vi "overwritePos.vi"(2 "overwrite angle":bool, 3 "Source":u16(ring) items=["Odometry", "Lidar"], 4 "lidarPosInput":cluster{"xPos":dbl, "yPos":dbl, "Theta":dbl}, 5 "odomPosInput":cluster{"xPos":dbl, "yPos":dbl, "Theta":dbl}) -> (1 "posOutput":cluster{"xPos":dbl, "yPos":dbl, "Theta":dbl})   [LabVIEW 2016]
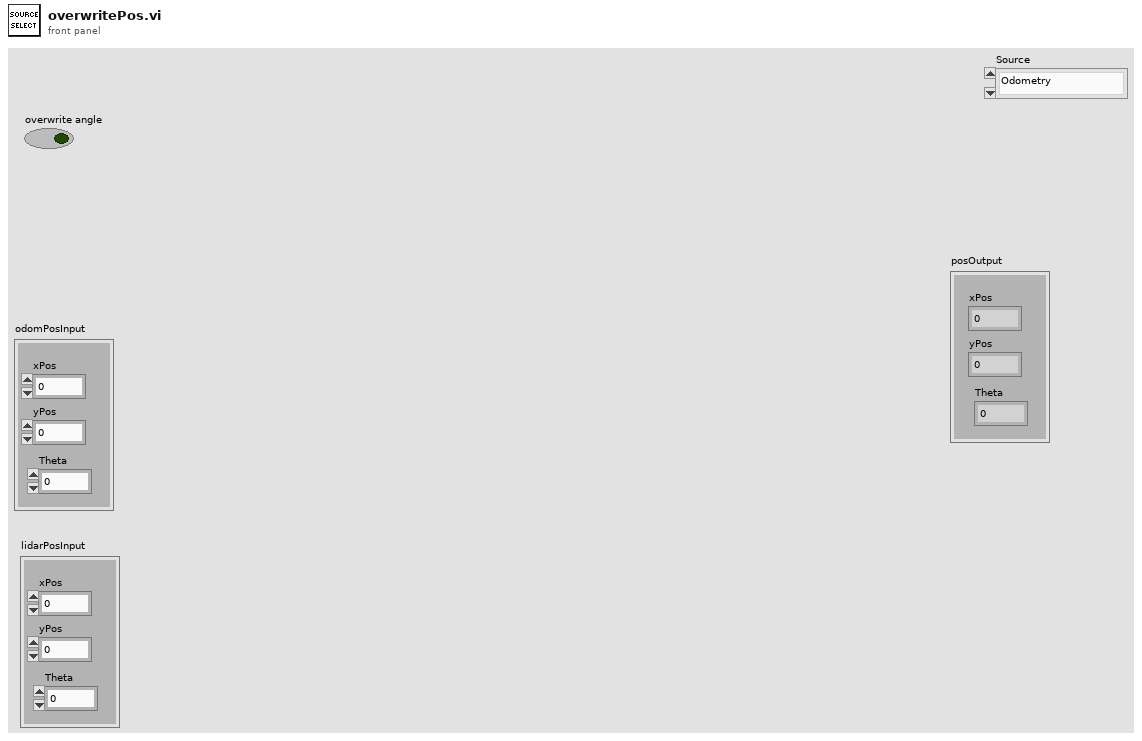
[diagram p1: front panel]
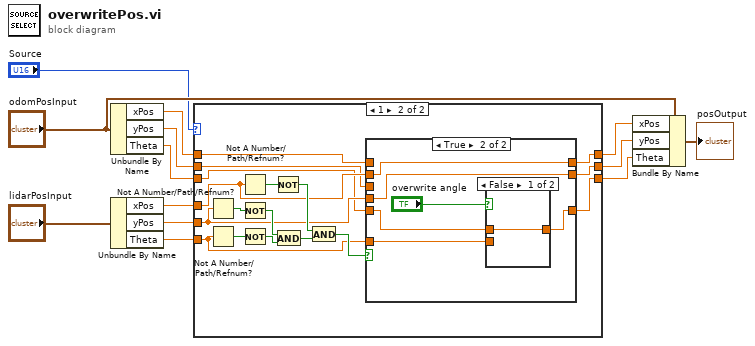
[diagram p0: block diagram]
diagram:
  n1 = Unbundle By Name("odomPosInput") -> ("xPos"=w5:dbl, "yPos"=w4:dbl, "Theta"=w1:dbl)
  n2 = Unbundle By Name("lidarPosInput") -> ("xPos"=w3:dbl, "yPos"=w7:dbl, "Theta"=w2:dbl)
  n3 = case shown="1" "Source" {
    tunnel: [w16 w25] -> w12
    tunnel: w5 -> [w16 w19]
    tunnel: [w15 w23] -> w11
    tunnel: w4 -> [w15 w18]
    tunnel: [w14 w21] -> w10
    tunnel: w1 -> [w14 w17]
    tunnel: w3 -> [_ w24]
    tunnel: w7 -> [_ w22]
    tunnel: w2 -> [_ w20]
    frame 0, Default {
    }
    frame 1 {
      n4 = Not A Number/Path/Refnum?(number/path/refnum=w22) -> (NaN/Path/Refnum?=w32:bool)
      n5 = Not A Number/Path/Refnum?(number/path/refnum=w20) -> (NaN/Path/Refnum?=w33:bool)
      n6 = Not A Number/Path/Refnum?(number/path/refnum=w24) -> (NaN/Path/Refnum?=w31:bool)
      n7 = Not(x=w32) -> (.not. x?=w30:bool)
      n8 = Not(x=w33) -> (.not. x?=w29:bool)
      n9 = Not(x=w31) -> (.not. x?=w27:bool)
      n10 = And(x=w30, y=w29) -> (x .and. y?=w28:bool)
      n11 = And(x=w27, y=w28) -> (x .and. y?=w26:bool)
      n12 = case shown="True" w26 {
        tunnel: [w36 w42] -> w25
        tunnel: w24 -> [_ w42]
        tunnel: [w35 w41] -> w23
        tunnel: w22 -> [_ w41]
        tunnel: [w34 w40] -> w21
        tunnel: w20 -> [_ w38]
        tunnel: w19 -> [w36 _]
        tunnel: w18 -> [w35 _]
        tunnel: w17 -> [w34 w39]
        frame False {
        }
        frame True {
          n13 = case shown="False" "overwrite angle" {
            tunnel: [w43 w44] -> w40
            tunnel: w38 -> [_ w44]
            tunnel: w39 -> [w43 _]
            frame False {
            }
            frame True {
            }
          }
        }
      }
    }
  }
  n14 = Bundle By Name(cluster="odomPosInput", "xPos"=w12, "yPos"=w11, "Theta"=w10) -> (→"posOutput":cluster{"xPos":dbl, "yPos":dbl, "Theta":dbl})
